vi "Express Servo Ard.vi"() -> ()   [LabVIEW 2015]
uses:
  <vilib>/rvi/Emulation/niFpgaGetClockAttributes.vi
  <vilib>/rvi/Emulation/niFpgaSctlEmulationGetInTimedLoop.vi
  <vilib>/rvi/Emulation/niFpgaEmulationReportErrorSimple.vi
  <vilib>/rvi/eio/common/nirviEmuTemplateMethod_errors.vi
  <vilib>/rvi/Emulation/niFpgaCriticalErrorInLSC.vi
  <vilib>/eio/EIONode/EIONode.xnode
panel:
  in  "Stop Button":bool
  in  "Servo 4":u16
  in  "Servo 3":u16
  in  "Servo 2":u16
  in  "Servo 1":u16
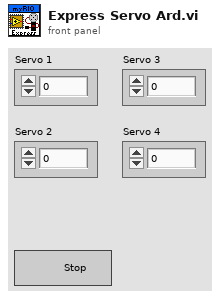
[diagram p1: front panel]
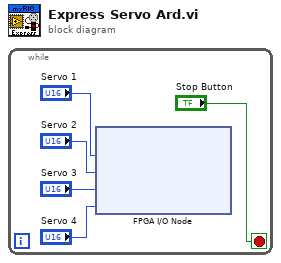
[diagram p0: block diagram]
diagram:
  n1 = while {
    stop <- "Stop Button" stop-if-true
    n2 = xnode "FPGA I/O Node"("ConnectorA/AO0"="Servo 1", "ConnectorA/AO1"="Servo 2", "ConnectorB/AO0"="Servo 3", "ConnectorB/AO1"="Servo 4") -> ()  [unwired: 4 in, 4 out]
  }
